vi "New Message.vi"(8 "error in (no error)":errorcluster, 10 "New Message":string, 11 "Communication Clients in":refnum<class "Communication Clients.lvclass">) -> (0 "error out":errorcluster, 3 "Communication Clients out":refnum<class "Communication Clients.lvclass">)   [LabVIEW 2017, in "Communication Clients.lvlib" / "Communication Clients.lvclass"]
uses:
  Communication Clients.lvclass
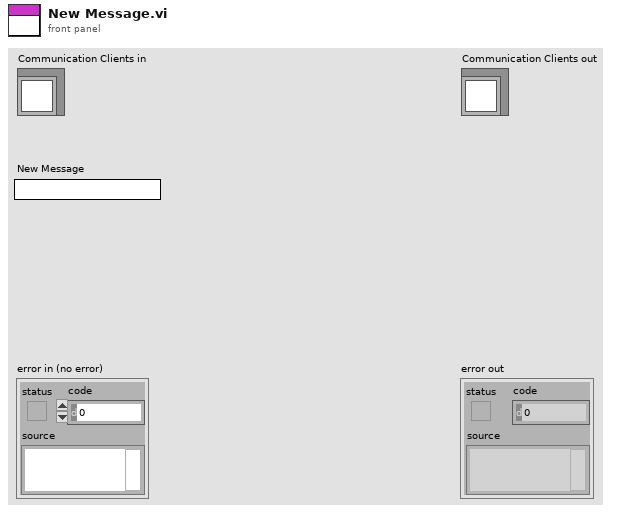
[diagram p1: front panel]
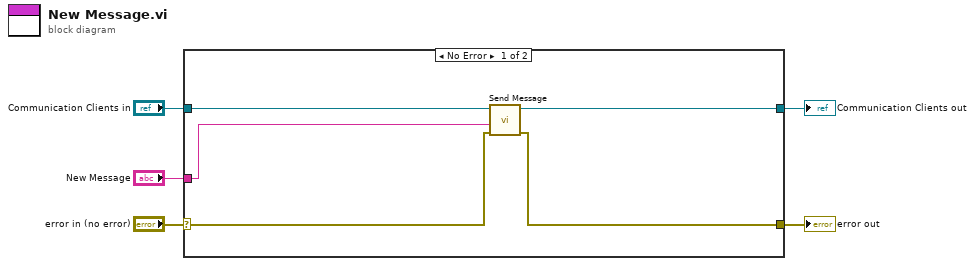
[diagram p0: block diagram]
diagram:
  n1 = case shown="No Error" "error in (no error)" {
    selector: "error in (no error)" -> [w7 w12]
    tunnel: [w6 w12] -> w4
    tunnel: [w9 w11] -> w2
    tunnel: "Communication Clients in" -> [w10 w11]
    tunnel: "New Message" -> [w8 _]
    frame No Error {
      n2 = call "Send Message.vi"("error in (no error)"=w7, "Message"=w8, "Communication Clients in"=w10) -> ("error out"=w6:errorcluster, "Communication Clients out"=w9:refnum<class "Communication Clients.lvclass">)  [unwired: 7 in]
    }
    frame Error {
    }
  }
  "error out" <- w4
  "Communication Clients out" <- w2
